vi "Teardown.vi"(8 "Error In":errorcluster, 10 "Temporary Directory":string, 11 "SFTP":refnum<class "SFTP.lvclass">) -> (0 "Error Out":errorcluster)   [LabVIEW 2018, in "Tests.lvlib" / "SFTP Directory.lvlib"]
uses:
  SFTP Directory.lvlib
  src/Toolkit/SFTP/SFTP.lvclass
  src/Toolkit/Session/Session.lvclass
  src/Toolkit/SSH/SSH.lvclass
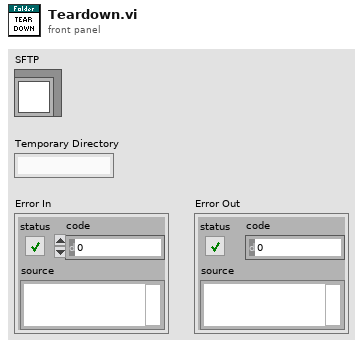
[diagram p1: front panel]
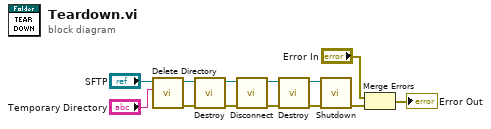
[diagram p0: block diagram]
diagram:
  n1 = call "Delete Directory.vi"("Remote Path"="Temporary Directory", "SFTP In"="SFTP") -> ("Error Out"=w2:errorcluster, "SFTP Out"=w3:refnum<class "SFTP.lvclass">)  [unwired: 8 in]
  n2 = call "Destroy.vi"("Error In"=w2, "SFTP"=w3) -> ("Error Out"=w13:errorcluster, "Session"=w5:refnum<class "Session.lvclass">)  [unwired: 8 in]
  n3 = call "Disconnect.vi"("Error In"=w13, "Session In"=w5) -> ("Error Out"=w12:errorcluster, "Sesssion Out"=w11:refnum<class "Session.lvclass">)  [unwired: 8 in]
  n4 = call "Destroy.vi"("Error In"=w12, "Session"=w11) -> ("Error Out"=w9:errorcluster, "SSH"=w8:refnum<class "SSH.lvclass">)  [unwired: 8 in]
  n5 = call "Shutdown.vi"("Error In"=w9, "SSH"=w8) -> ("Error Out"=w10:errorcluster)  [unwired: 9 in]
  n6 = Merge Errors("Error In", w10) -> (→"Error Out":errorcluster)
